vi "const_bias_conductance.vi"() -> ()   [LabVIEW 2010]
uses:
  <vilib>/Utility/file.llb/Write To Spreadsheet File (DBL).vi
  <userlib>/Nanonis Prog Interface V5/Nanonis Prog Interface.lvlib
panel:
  in  "Settling Time between gate":u32
  in  "Wait Time between AVG":i32
  out "Input 2 (V)":sgl
  out "XY Graph":cluster{dbl[], dbl[]}(graph)
  in  "Averages":i32
  out "Current Gate Voltage (V)":dbl
  in  "Stop":bool
  in  "Increment Gate (V)":dbl
  in  "End Gate (V)":dbl
  in  "Start Gate (V)":dbl
  in  "Filename":string
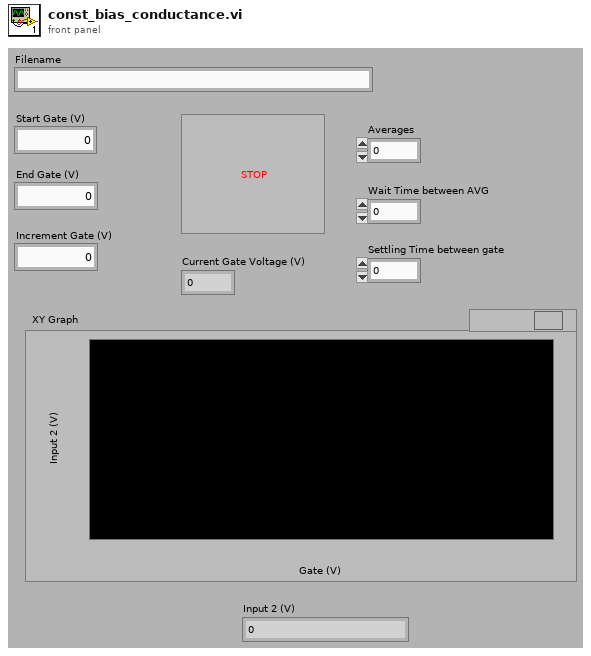
[diagram p1: front panel]
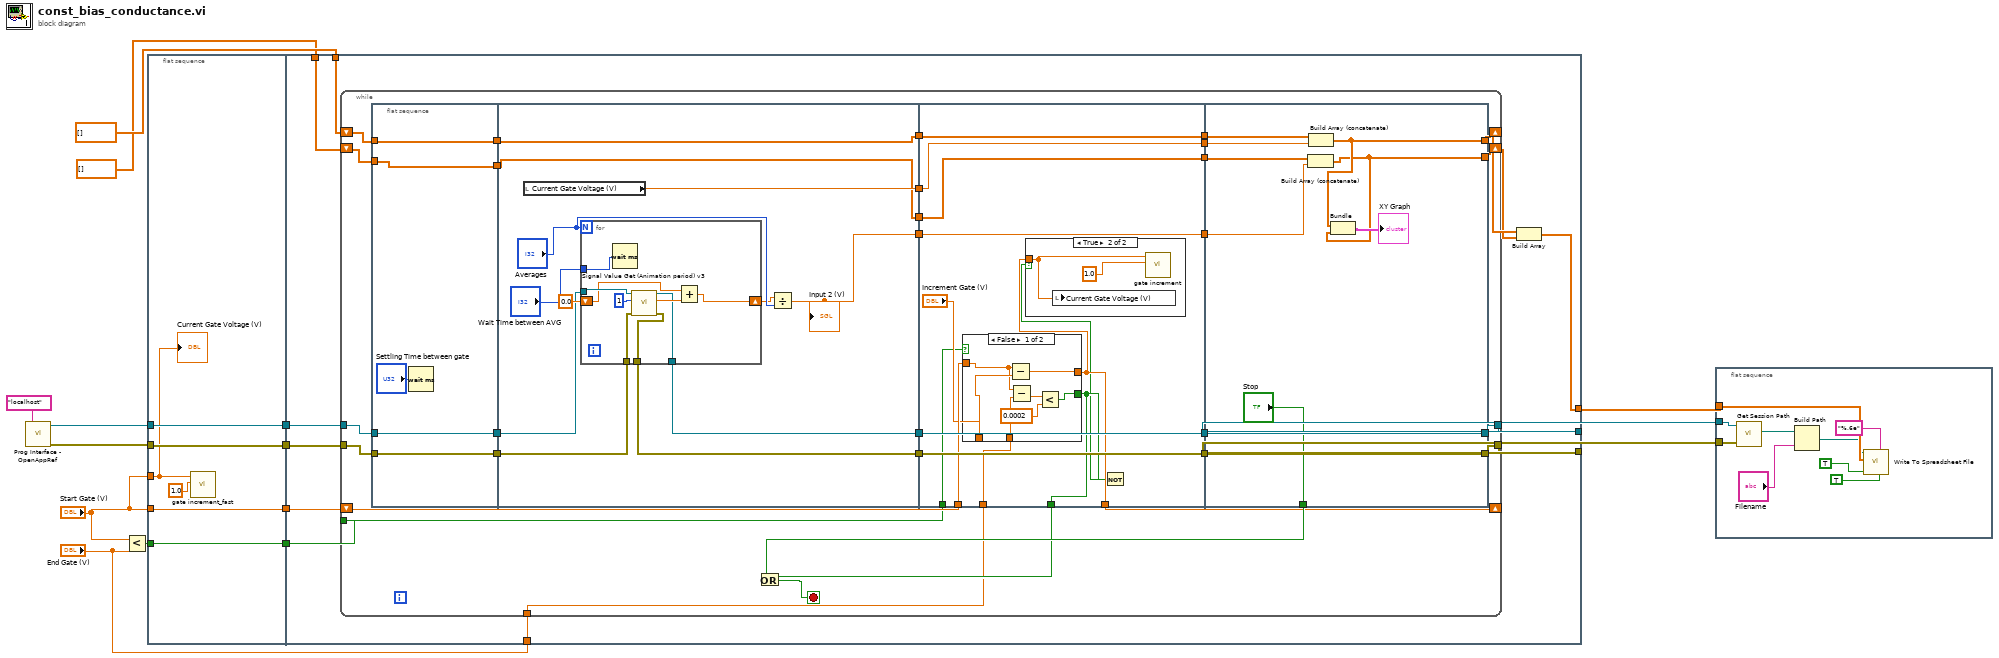
[diagram p0: block diagram]
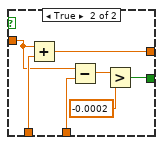
[diagram p2: hidden frame]
diagram:
  n1 = call <userlib>:"Prog Interface - OpenAppRef.vi"("Machine name (local machine IP)"="localhost" ("machine name (localhost)")) -> ("Error out"=w4:errorcluster, "Application reference"=w5:refnum<vi>)  [unwired: 5 in]
  n2 = Less?(x="Start Gate (V)", y="End Gate (V)") -> (x < y?=w12:bool)
  n3 = flat-sequence {
    tunnel: "Start Gate (V)" -> [w18]
    tunnel: w12 -> [w19]
    tunnel: w5 -> [w20]
    tunnel: w4 -> [w21]
    tunnel: [w21] -> w11
    tunnel: [w20] -> w10
    tunnel: [w19] -> w9
    tunnel: [w18] -> w8
    tunnel: "Start Gate (V)" -> [w16]
    tunnel: [w31] -> w14
    tunnel: [w30] -> w13
    tunnel: w11 -> [w33]
    tunnel: w10 -> [w32]
    tunnel: w9 -> [w29]
    tunnel: w8 -> [w28]
    tunnel: "End Gate (V)" -> [w27]
    tunnel: [w24] -> w3
    tunnel: dbl[] [] -> [w23]
    tunnel: dbl[] [] -> [w22]
    frame #0 {
      n4 = call "gate increment_fast.vi"("Increment"=1.0, "Gate Voltage"=w16) -> ()  [unwired: 10 in]
      "Current Gate Voltage (V)" <- w16
    }
    frame #1 {
      n5 = while {
        tunnel: w33 -> [w64]
        tunnel: w32 -> [w63]
        tunnel: [w62] -> w31
        tunnel: [w61] -> w30
        tunnel: w29 -> [w50]
        shift-right: [w54] -> _
        shift-left: w28 -> [w52]
        tunnel: w27 -> [w51]
        shift-right: [w44] -> w26
        shift-left: w23 -> [w43]
        shift-right: [w41] -> w25
        shift-left: w22 -> [w36]
        stop <- w55 stop-if-true
        n6 = flat-sequence {
          tunnel: w63 -> [w68]
          tunnel: w64 -> [w69]
          tunnel: [w69] -> w58
          tunnel: [w68] -> w57
          tunnel: w43 -> [w66]
          tunnel: w36 -> [w67]
          tunnel: [w67] -> w37
          tunnel: [w66] -> w35
          tunnel: w58 -> [w81]
          tunnel: w57 -> [w77]
          tunnel: [w76] -> w49
          tunnel: [w75] -> w48
          tunnel: [w74] -> w47
          tunnel: [w72] -> w40
          tunnel: [w73] -> w39
          tunnel: w37 -> [w72]
          tunnel: w35 -> [w71]
          tunnel: [w71] -> w34
          tunnel: [w103] -> w60
          tunnel: [w102] -> w59
          tunnel: [w101] -> w54
          tunnel: [w100] -> w53
          tunnel: w52 -> [w99]
          tunnel: w51 -> [w97]
          tunnel: w50 -> [w96]
          tunnel: w49 -> [w102]
          tunnel: w48 -> [w103]
          tunnel: w47 -> [w94]
          tunnel: [w94] -> w46
          tunnel: [w93] -> w45
          tunnel: [w92] -> w42
          tunnel: w40 -> [w92]
          tunnel: w39 -> [w91]
          tunnel: [w91] -> w38
          tunnel: w34 -> [w93]
          tunnel: [w128] -> w62
          tunnel: [w129] -> w61
          tunnel: w60 -> [w129]
          tunnel: w59 -> [w128]
          tunnel: ["Stop"] -> w56
          tunnel: [w121] -> w44
          tunnel: w46 -> [w126]
          tunnel: w45 -> [w125]
          tunnel: w42 -> [w124]
          tunnel: [w120] -> w41
          tunnel: w38 -> [w123]
          frame #0 {
            n7 = Wait (ms)(milliseconds to wait="Settling Time between gate") -> ()  [unwired: 1 out]
          }
          frame #1 {
            n8 = local read "Current Gate Voltage (V)"() -> (w74:dbl)
            n9 = for {
              N: "Averages" -> [_]
              tunnel: w77 -> [w89]
              tunnel: w81 -> [w88]
              shift-right: [w85] -> w79
              shift-left: sgl 0.0 -> [w86]
              tunnel: [w84] -> w76
              tunnel: [w83] -> w75
              tunnel: "Wait Time between AVG" -> [w82]
              n10 = Wait (ms)(milliseconds to wait=w82) -> ()  [unwired: 1 out]
              n11 = call <userlib>:"Signal Value Get (Animation period) v3.vi"("error in (no error)"=w88, "Signal index (0-127)"=i8 1, "Application ref in"=w89) -> ("error out"=w83:errorcluster, "Signal value"=w87:sgl, "Application ref out"=w84:refnum<vi>)  [unwired: 5 in]
              n12 = Add(x=w86, y=w87) -> (x+y=w85:sgl)
            }
            n13 = Divide(x=w79, y="Averages") -> (x/y=w73:sgl)
            "Input 2 (V)" <- w73
          }
          frame #2 {
            n14 = case shown="False" w96 {
              tunnel: w99 -> [w108 w114]
              tunnel: "Increment Gate (V)" -> [w109 w117]
              tunnel: [w110 w116] -> w101
              tunnel: w97 -> [w107 w115]
              tunnel: [w105 w113] -> w100
              frame False {
                n15 = Subtract(x=w108, y=w109) -> (x-y=w110:dbl)
                n16 = Subtract(x=w108, y=w107) -> (x-y=w106:dbl)
                n17 = Less?(x=w106, y=0.0002) -> (x < y?=w105:bool)
              }
              frame True {
                n18 = Add(x=w114, y=w117) -> (x+y=w116:dbl)
                n19 = Subtract(x=w114, y=w115) -> (x-y=w112:dbl)
                n20 = Greater?(x=w112, y=-0.0002) -> (0:w113:bool)
              }
            }
            n21 = Not(x=w100) -> (.not. x?=w95:bool)
            n22 = case shown="True" w95 {
              tunnel: w101 -> [_ w118]
              frame False {
              }
              frame True {
                n23 = local write "Current Gate Voltage (V)"(w118) -> ()
                n24 = call "gate increment.vi"("Increment"=1.0, "Gate Voltage"=w118) -> ()  [unwired: 8 in, 2 out]
              }
            }
          }
          frame #3 {
            n25 = Build Array (concatenate)(w124, w123) -> (w120:dbl[])
            n26 = Build Array (concatenate)(w125, w126) -> (w121:dbl[])
            n27 = Bundle(w121, w120) -> (→"XY Graph":cluster{dbl[], dbl[]})  [unwired: 1 in]
          }
        }
        n28 = Or(x=w53, y=w56) -> (x .or. y?=w55:bool)
      }
      n29 = Build Array(w26, w25) -> (w24:dbl[][])
    }
  }
  n30 = flat-sequence {
    tunnel: w14 -> [w135]
    tunnel: w13 -> [w134]
    tunnel: w3 -> [w136]
    frame #0 {
      n31 = call <userlib>:"Get Session Path.vi"("error in (no error)"=w134, "Application ref in"=w135) -> ("Session path"=w131:path)  [unwired: 7 in, 2 out]
      n32 = Build Path(base path=w131, name or relative path="Filename") -> (appended path=w133:path)
      n33 = call-poly <vilib>:"Write To Spreadsheet File.vi"("transpose? (no:F)"=TRUE ("append to file? (new file:F)"), "format (%.3f)"="%.6e", "append to file? (new file:F)"=TRUE, "2D data"=w136, "file path (dialog if empty)"=w133) -> ()  [unwired: 3 in, 1 out]
    }
  }
